vi "TCP Msg Read.vi"(0 "connection ID":refnum<k5>, 1 "timeout ms (25000)":i32=25000, 5 "error in":errorcluster) -> (12 "Timed Out?":bool, 14 "connection ID out":refnum<k5>, 15 "Command Type":i32, 17 "Msg Data":string, 18 "Msg Head":string, 19 "error out":errorcluster)   [LabVIEW 2014]
doc: "Reads an incoming package of data from a remote host via TCP/IP. This VI parses the package and extracts the data name and type as described in the meta data.\n\nFor the package to be parsed correctly, the meta data must be consistent in both the sender and the receiver. The data is packaged based on the existing meta data on the sender. Inconsistent meta data will result in inconsistent data parsing.\nUse the \"Read Meta\" and \"Write Meta\" VIs to ensure that both client and server have the same meta data.\n\nThe data is returned as a string. It is the responsibility of the user to cast it to the appropriate type before usage."
panel:
  out "element":i32
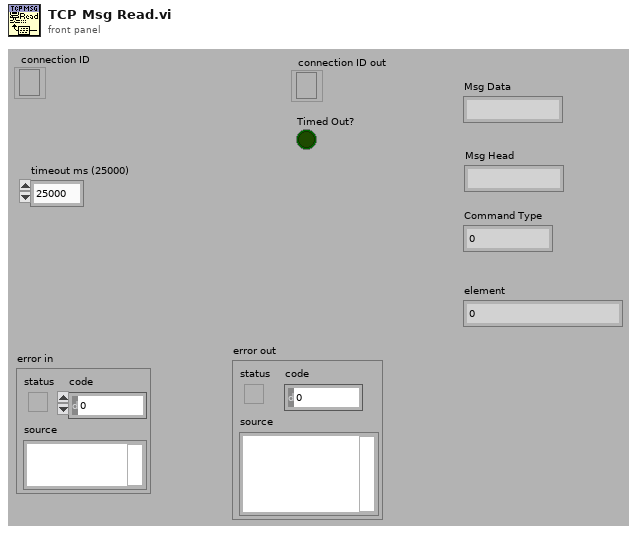
[diagram p1: front panel]
types:
  T1 = enum16{"big-endian, network order", "native, host order", "little-endian"}
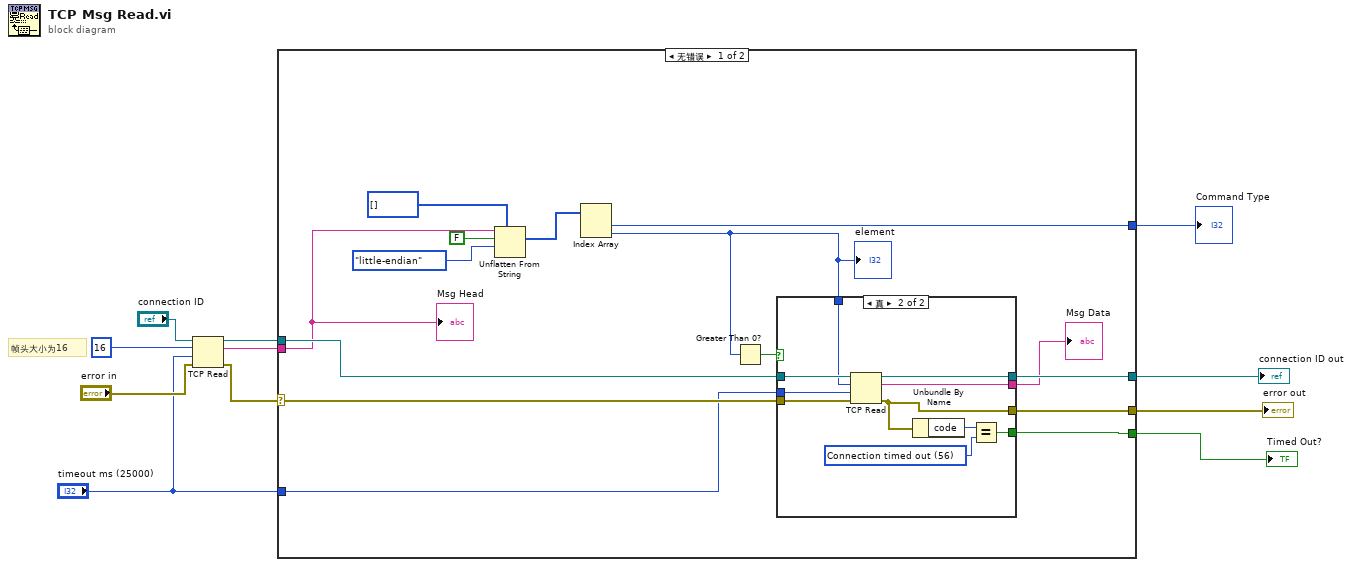
[diagram p0: block diagram]
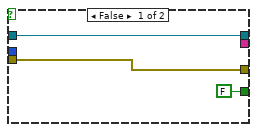
[diagram p2: hidden frame]
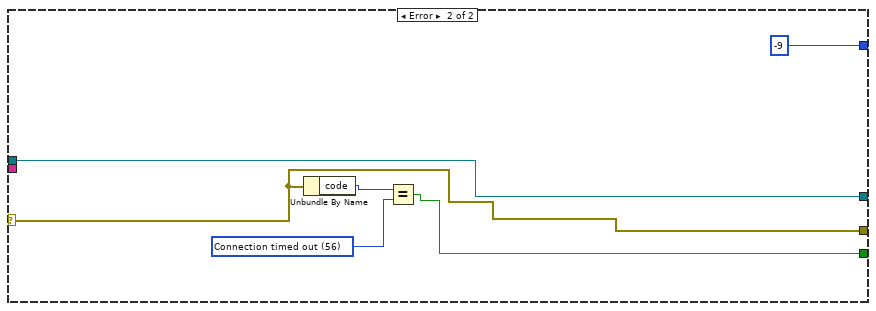
[diagram p3: hidden frame]
diagram:
  # "帧头大小为16"
  n1 = TCP Read(connection ID="connection ID", bytes to read=16, error in (no error)="error in", 9:"timeout ms (25000)") -> (connection ID out=w7:refnum<k5>, data out=w8:string, error out=w5:errorcluster)  [unwired: 1 out]
  n2 = case shown="无错误" w5 {
    selector: w5 -> [w25 w42]
    tunnel: w8 -> [w18 _]
    tunnel: w7 -> [w26 w45]
    tunnel: "timeout ms (25000)" -> [w20 _]
    tunnel: [w24 w45] -> w4
    tunnel: [w23 w42] -> w3
    tunnel: [w22 w41] -> w2
    tunnel: [w13 -9] -> w1
    frame No Error {
      n3 = Unflatten From String(type=i32[] [], binary string=w18, data includes array or string size? (T)=FALSE, byte order (0:big-endian, network order)=T1."little-endian") -> (value=w14:i32[])  [unwired: 1 in, 2 out]
      n4 = Index Array(array=w14) -> (element #1=w13:i32, element #2=w12:i32)  [unwired: 2 in]
      "element" <- w12
      n5 = Greater Than 0?(x=w12) -> (x > 0?=w19:bool)
      n6 = case shown="真" w19 {
        tunnel: w26 -> [w29 w39]
        tunnel: w25 -> [w28 w38]
        tunnel: [w29 w37] -> w24
        tunnel: [w28 w34] -> w23
        tunnel: [FALSE w33] -> w22
        tunnel: [_ w32] -> w21
        tunnel: w20 -> [_ w31]
        tunnel: w12 -> [_ w30]
        frame False {
        }
        frame True {
          w35 = 56 items=["No Error", "Argument Error", "Memory Full", "Out of Zone", "End of File", "File Already Open", "Generic File IO Error", "File Not Found", "File Permission Error", "Disk Full", "Duplicate Path", "Too Many Files Open", "Not Enabled", "Resource File Not Found", "Cannot Add Resource", "Resource Not Found", "Image Not Found", "Image Memory Error", "Pen Does Not Exist", "Config Bad Type", "Config Token Not Found", "Config Parse Error", "Config Memory Error", "Bad External Code Format", "Bad External Code Offset", "External Code Not Present", "Null Window", "Destroy Window Mixup", "Null Menu", "Print Aborted", "Bad Print Record", "Print Driver Error", "Windows Error During Print", "Memory Error During Print", "Print Dialog Error", "Generic Print Error", "Invalid Device Refnum", "Device Not Found", "Device Parameter Error", "Device Unit Error", "Can't Open Device", "Device Call Aborted", "Generic Error", "Cancelled By User", "Object ID Too Low", "Object ID Too High", "Object Not In Heap", "Unknown Heap", "Bad DefProc ID", "DefProc Not In Table", "Message Out Of Range", "Null Method", "Unknown Message", "Manager Call Not Supported", "Bad address", "Connection In progress", "Connection timed out", "Connection is already in progress", "Network attribute not supported", "Network error", "Address in use", "System out of memory", "Connection aborted", "Connection refused", "Connection is not connected", "Connection is already connected", "Connection closed", "Initialize error (interapplication manager)", "Bad occurrence", "Wait on unbound occurrence handler", "Occurrence queue overflow", "Bad path", "Semaphore not signaled", "Unrecognized type (interapplication manager)"] ("1st Error to Convert")
          n7 = TCP Read(connection ID=w39, bytes to read=w30, error in (no error)=w38, 9:w31) -> (connection ID out=w37:refnum<k5>, data out=w32:string, error out=w34:errorcluster)  [unwired: 1 out]
          n8 = Unbundle By Name(w34) -> ("code"=w36:i32)
          n9 = Equal?(x=w36, y=w35) -> (x = y?=w33:bool)
        }
      }
      "Msg Data" <- w21
      "Msg Head" <- w18
    }
    frame Error {
      w43 = 56 items=["No Error", "Argument Error", "Memory Full", "Out of Zone", "End of File", "File Already Open", "Generic File IO Error", "File Not Found", "File Permission Error", "Disk Full", "Duplicate Path", "Too Many Files Open", "Not Enabled", "Resource File Not Found", "Cannot Add Resource", "Resource Not Found", "Image Not Found", "Image Memory Error", "Pen Does Not Exist", "Config Bad Type", "Config Token Not Found", "Config Parse Error", "Config Memory Error", "Bad External Code Format", "Bad External Code Offset", "External Code Not Present", "Null Window", "Destroy Window Mixup", "Null Menu", "Print Aborted", "Bad Print Record", "Print Driver Error", "Windows Error During Print", "Memory Error During Print", "Print Dialog Error", "Generic Print Error", "Invalid Device Refnum", "Device Not Found", "Device Parameter Error", "Device Unit Error", "Can't Open Device", "Device Call Aborted", "Generic Error", "Cancelled By User", "Object ID Too Low", "Object ID Too High", "Object Not In Heap", "Unknown Heap", "Bad DefProc ID", "DefProc Not In Table", "Message Out Of Range", "Null Method", "Unknown Message", "Manager Call Not Supported", "Bad address", "Connection In progress", "Connection timed out", "Connection is already in progress", "Network attribute not supported", "Network error", "Address in use", "System out of memory", "Connection aborted", "Connection refused", "Connection is not connected", "Connection is already connected", "Connection closed", "Initialize error (interapplication manager)", "Bad occurrence", "Wait on unbound occurrence handler", "Occurrence queue overflow", "Bad path", "Semaphore not signaled", "Unrecognized type (interapplication manager)"] ("1st Error to Convert")
      n10 = Unbundle By Name(w42) -> ("code"=w44:i32)
      n11 = Equal?(x=w44, y=w43) -> (x = y?=w41:bool)
    }
  }
  "error out" <- w3
  "connection ID out" <- w4
  "Timed Out?" <- w2
  "Command Type" <- w1
